vi "getContext.vi"(0 "session in":refnum<class "niInstr FIFO Register Bus v1 Host.lvclass">, 5 "instance":u8, 11 "error in":errorcluster) -> (4 "session out":refnum<class "niInstr FIFO Register Bus v1 Host.lvclass">, 6 "ScalingAndLimitsContext":refnum<class "niInstr Instruction Framework Context v1 Host.lvclass">, 15 "error out":errorcluster)   [LabVIEW 2017, in "ScaleAndLimitInterface.lvlib"]
uses:
  ScaleAndLimitInterface.lvlib
  <instrlib>/_niInstr/Instruction Framework/v1/Host/Instruction Framework Context/niInstr Instruction Framework Context v1 Host.lvclass
  <instrlib>/_niInstr/FIFO Register Bus/v1/Host/niInstr FIFO Register Bus v1 Host.lvclass
  C:/Program Files (x86)/National Instruments/LabVIEW 2017/instr.lib/_niInstr/Instruction Framework/v1/Host/Instruction Target/niInstr Instruction Target v1 Host.lvclass
  <instrlib>/_niInstr/Instruction Framework/v1/Host/Subsystem Map/Private/Lookup Single Context.vi
  <instrlib>/_niInstr/Instruction Framework/v1/Host/Subsystem Map/niInstr Subsystem Map v1 Host.lvclass
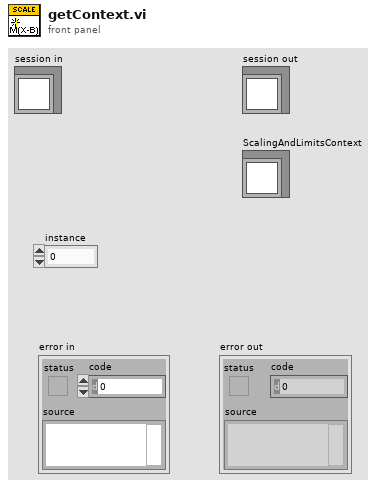
[diagram p1: front panel]
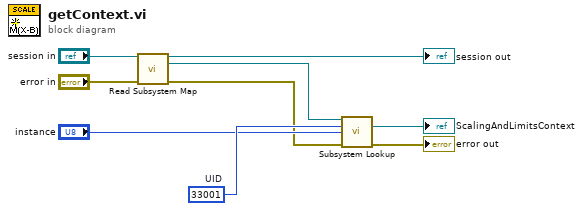
[diagram p0: block diagram]
diagram:
  w9 = u16 33001  # UID
  n1 = call <instrlib>:"Read Subsystem Map.vi"("instruction target in"="session in", "error in"="error in") -> ("instruction target out"=→"session out":refnum<class "niInstr FIFO Register Bus v1 Host.lvclass">, "subsystem map"=w3:refnum<class "niInstr Subsystem Map v1 Host.lvclass">, "error out"=w1:errorcluster)  [unwired: 11 in]
  n2 = call-poly <instrlib>:"Subsystem Lookup.vi"("subsystem map in"=w3, "UID"=w9, "instance"="instance", "error in"=w1) -> ("context"=→"ScalingAndLimitsContext":refnum<class "niInstr Instruction Framework Context v1 Host.lvclass">, "error out"=→"error out":errorcluster)  [unwired: 8 in, 2 out]
